vi "AdaptToInputs.vi"(3 "Term Types":T1, 4 "XRef":refnum<vi>, 5 "State In":T5) -> (0 "Reply":string[](array[string]), 2 "State Out":T5)   [LabVIEW 2018, in "OpenG Remove Duplicates from 1 D Array.xnode"]
uses:
  OpenG Remove Duplicates from 1 D Array.xnode
  State.ctl
  <vilib>/XNodeSupport/XNodeTermTypeIDPairs.ctl
  <vilib>/XNodeSupport/XNodeTermTypeIDPair.ctl
  <vilib>/XNodeSupport/XNodeType.ctl
  <vilib>/XNodeSupport/XNodeString.ctl
  <userlib>/_LAVAcr/Scripting Tools/XNode Support/TypeDefs/Array element Tests.ctl
  <userlib>/_LAVAcr/Scripting Tools/XNode Support/Find term type by ID_type.vi
  <userlib>/_LAVAcr/Scripting Tools/XNode Support/XNode Support.lvlib
  <vilib>/XNodeSupport/NI_XNodeSupport.lvlib
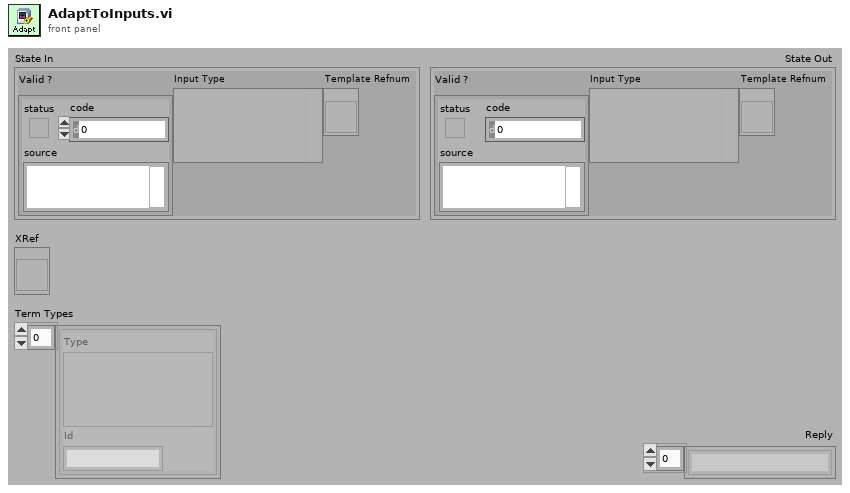
[diagram p1: front panel]
types:
  T1 = typedef "NI_XNodeSupport.lvlib/XNodeTermTypeIDPairs.ctl" = T2[]
  T2 = typedef "NI_XNodeSupport.lvlib/XNodeTermTypeIDPair.ctl" = cluster{"Type":T3, "Id":T4}
  T3 = typedef "NI_XNodeSupport.lvlib/XNodeType.ctl" = variant
  T4 = typedef "NI_XNodeSupport.lvlib/XNodeString.ctl" = string
  T5 = typedef "OpenG Remove Duplicates from 1 D Array.xnode/State.ctl" = cluster{"Valid ?":errorcluster, "Input Type":variant, "Template Refnum":refnum<vi>}
  T6 = typedef "Scripting Tools.lvlib/XNode Support.lvlib/Array element Tests.ctl" = enum16{"Any Element", "Numeric", "Integer", "Float", "Complex", "Boolean", "String", "Sortable"}
  T7 = enum16{"No Check", "At Least n dimensions", "Exactly N Dimensions"}
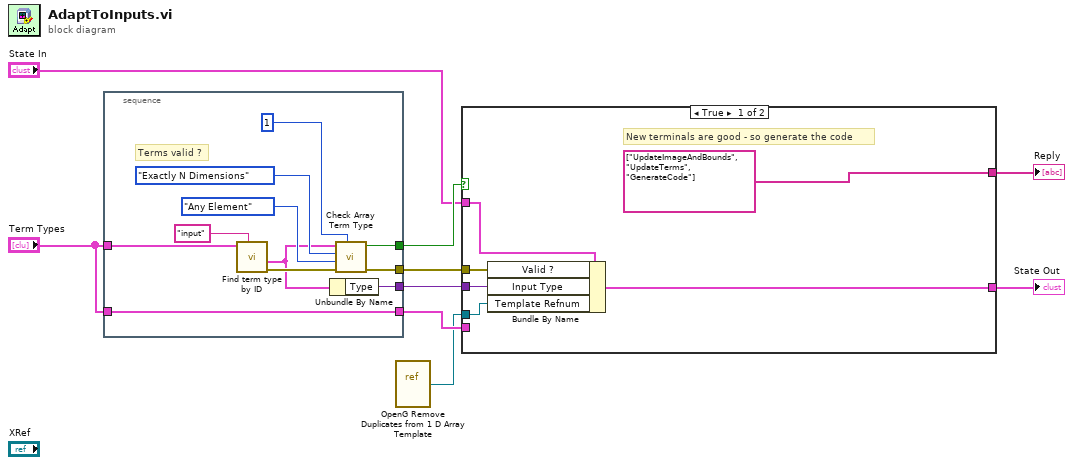
[diagram p0: block diagram]
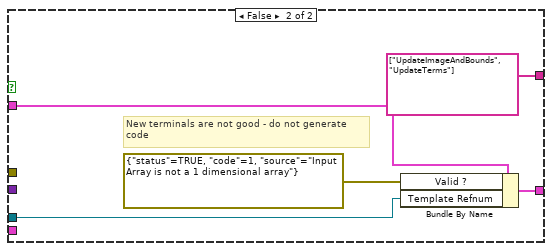
[diagram p2: hidden frame]
diagram:
  n1 = stacked-sequence {
    tunnel: "Term Types" -> [w20]
    tunnel: [w20] -> w8
    tunnel: [w13] -> w9
    tunnel: "Term Types" -> [w19]
    tunnel: [w11] -> w3
    tunnel: [w10] -> w2
    frame #0 {
      # "Terms valid ?"
      n2 = call-poly <userlib>:"Find term type by ID.vi"("Search ID"="input", "Term Types"=w19) -> ("error out"=w17:errorcluster, "Term Type"=w12:T2)  [unwired: 1 in, 7 out]
      n3 = Unbundle By Name(w12) -> ("Type"=w11:T3)
      n4 = call <userlib>:"Check Array Term Type.vi"("Dimensions Required"=1, "error in (no error)"=w17, "Element Check"=Array_element_Tests."Any Element", "Dimension Check"=T7."Exactly N Dimensions", "Term Type"=w12) -> ("error out"=w10:errorcluster, "Is Good ?"=w13:bool)  [unwired: 5 out]
    }
  }
  n5 = vi-ref "OpenG Remove Duplicates from 1 D Array Template.vi"() -> (w1:refnum<vi>)
  n6 = case shown="True" w9 {
    tunnel: w8 -> [_ _]
    tunnel: "State In" -> [w26 w31]
    tunnel: [w25 w29] -> w6
    tunnel: [string[] ["UpdateImageAndBounds", "UpdateTerms", "GenerateCode"] ("Reply") string[] ["UpdateImageAndBounds", "UpdateTerms"] ("Reply")] -> w5
    tunnel: w3 -> [w23 _]
    tunnel: w2 -> [w22 _]
    tunnel: w1 -> [w21 w27]
    frame True {
      # "New terminals are good - so generate the code"
      n7 = Bundle By Name(cluster=w26, "Valid ?"=w22, "Input Type"=w23, "Template Refnum"=w21) -> (w25:T5)
    }
    frame False {
      # "New terminals are not good - do not generate\ncode"
      n8 = Bundle By Name(cluster=w31, "Valid ?"=errorcluster {"status"=TRUE, "code"=1, "source"="Input Array is not a 1 dimensional array"}, "Template Refnum"=w27) -> (w29:T5)
    }
  }
  "Reply" <- w5
  "State Out" <- w6
